vi "Wait Until Cancelled or Complete.vi"(6 "done channel":T1, 8 "error in (no error)":errorcluster, 9 "ms polling interval":i32=100, 11 "measure call context in":refnum<class "Measure Call Context.lvclass">) -> (0 "error out":errorcluster, 3 "measure call context out":refnum<class "Measure Call Context.lvclass">)   [LabVIEW 2025, in "WorkflowDO.lvclass"]
doc: "Monitor for cancellation and abort the measurement if a cancellation request is received before the measurement completes normally."
uses:
  WorkflowDO.lvclass
  <vilib>/Plug-In SDKs/Measurements/Measure Call Context/Measure Call Context.lvclass
  <extravilib>/ChannelInstances/Event Messenger-bool/))Channel.ctl
  <extravilib>/ChannelInstances/Event Messenger-bool/))Channel.vi
  WorkflowDO.lvclass/WorkflowDO.ctl
  <extravilib>/ChannelInstances/Event Messenger-bool.lvlib
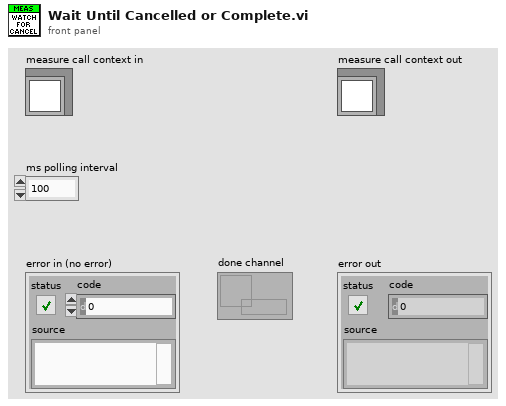
[diagram p1: front panel]
types:
  T1 = typedef "Event Messenger-bool.lvlib/))Channel.ctl" = refnum<queue>
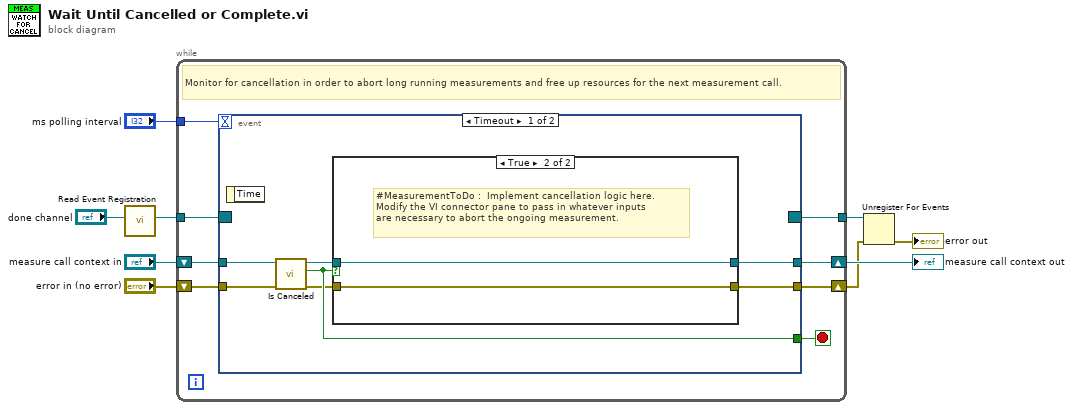
[diagram p0: block diagram]
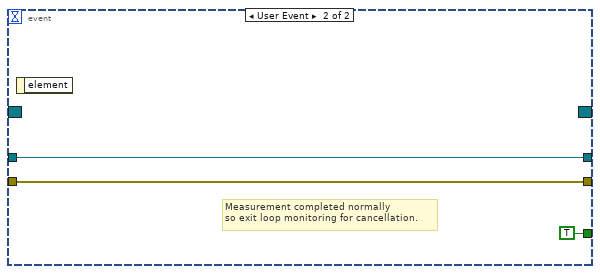
[diagram p3: hidden frame]
diagram:
  n1 = call <extravilib>:"Read Event Registration.vi"("channel"="done channel") -> ("event registration refnum"=w5:refnum<event-registration>)  [unwired: 10 in]
  n2 = while {
    shift-right: [w16] -> w9
    shift-left: "measure call context in" -> [w17]
    shift-right: [w13] -> w2
    shift-left: "error in (no error)" -> [w14]
    tunnel: w5 -> [w12]
    tunnel: "ms polling interval" -> [w11]
    tunnel: [w10] -> w3
    stop <- w15 stop-if-true
    # "Monitor for cancellation in order to abort long running measurements and free up resources for the next measurement call."
    n3 = event shown="[0] Timeout" {
      selector: w12 -> [_ _]
      dyn-events: [_ _] -> w10
      timeout: w11 -> [_ _]
      tunnel: w17 -> [w24 w29]
      tunnel: [w23 w29] -> w16
      tunnel: [w22 TRUE ("is canceled?")] -> w15
      tunnel: w14 -> [w21 w30]
      tunnel: [w20 w30] -> w13
      event Timeout {
        n4 = event-data() -> ()  [unwired: 1 in, 1 out]
        n5 = call <vilib>:"Is Canceled.vi"("error in"=w21, "measure call context in"=w24) -> ("error out"=w19:errorcluster, "is canceled?"=w22:bool, "measure call context out"=w18:refnum<class "Measure Call Context.lvclass">)  [unwired: 7 in]
        n6 = case shown="True" w22 {
          tunnel: w19 -> [w26 w27]
          tunnel: w18 -> [w25 w28]
          tunnel: [w26 w27] -> w20
          tunnel: [w25 w28] -> w23
          frame False {
          }
          frame True {
            # "#MeasurementToDo :  Implement cancellation logic here. \nModify the VI connector pane to pass in whatever inputs \nare necessary to abort the ongoing measurement."
          }
        }
      }
      event User Event {
        # "Measurement completed normally\nso exit loop monitoring for cancellation."
        n7 = event-data() -> ()  [unwired: 1 in, 1 out]
      }
    }
  }
  "measure call context out" <- w9
  n8 = Unregister For Events(event registration refnum=w3, error in=w2) -> (error out=→"error out":errorcluster)
